vi "aim.vi"() -> (0 "rate":dbl)   [LabVIEW 2011]
doc: "Aims the turret at the selected target."
uses:
  vision data.ctl
  fg_typedef.ctl
  <vilib>/addons/control/pid/pid.llb/PID (DBL).vi
  <vilib>/addons/control/pid/NI_PID_pid.lvlib
  <vilib>/addons/control/pid/pid.llb/PID Control Input Filter (DBL).vi
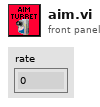
[diagram p1: front panel]
types:
  T1 = typedef "fg_typedef.ctl" = enum16{"Get", "Set"}
  T2 = typedef "vision data.ctl" = cluster{"x":dbl, "y":dbl, "area":dbl, "width":dbl, "height":dbl}
  T3 = cluster{"x":bool, "y":bool, "area":bool, "width":bool, "height":bool}
  T4 = typedef "WPI_EncoderDevRef.ctl" = cluster{"DevStatus":errorcluster, "EncoderIndex":T5, "CounterIndex":T6, "DistancePerCount":dbl, "Decoding Type":T7}
  T5 = typedef "FPGA_EncoderIdx.ctl" = enum8{"Enc 0", "Enc 1", "Enc 2", "Enc 3", "Invalid"}
  T6 = typedef "FPGA_CounterCtrSystemIndex.ctl" = enum8{"Ctr 0", "Ctr 1", "Ctr 2", "Ctr 3", "Ctr 4", "Ctr 5", "Ctr 6", "Ctr 7", "Invalid"}
  T7 = typedef "WPI_EncoderType.ctl" = enum16{"1x", "2x", "4x"}
  T8 = typedef "WPI_JoystickDevRef.ctl" = cluster{"Device":T9}
  T9 = typedef "WPI_JoystickDeviceEnum.ctl" = enum16{"USB 1", "USB 2", "USB 3", "USB 4", "Kinect 1", "Kinect 2"}
  T10 = cluster{"axis 1 (x)":dbl, "axis 2 (y)":dbl, "axis 3 (throttle)":dbl, "axis 4":dbl, "axis 5":dbl, "axis 6":dbl}
  T11 = cluster{"proportional gain (Kc)":dbl, "integral time (Ti, min)":dbl, "derivative time (Td, min)":dbl}
  T12 = cluster{dbl, "integral time (Ti, min)":dbl, "integral time (Ti, min)":dbl}
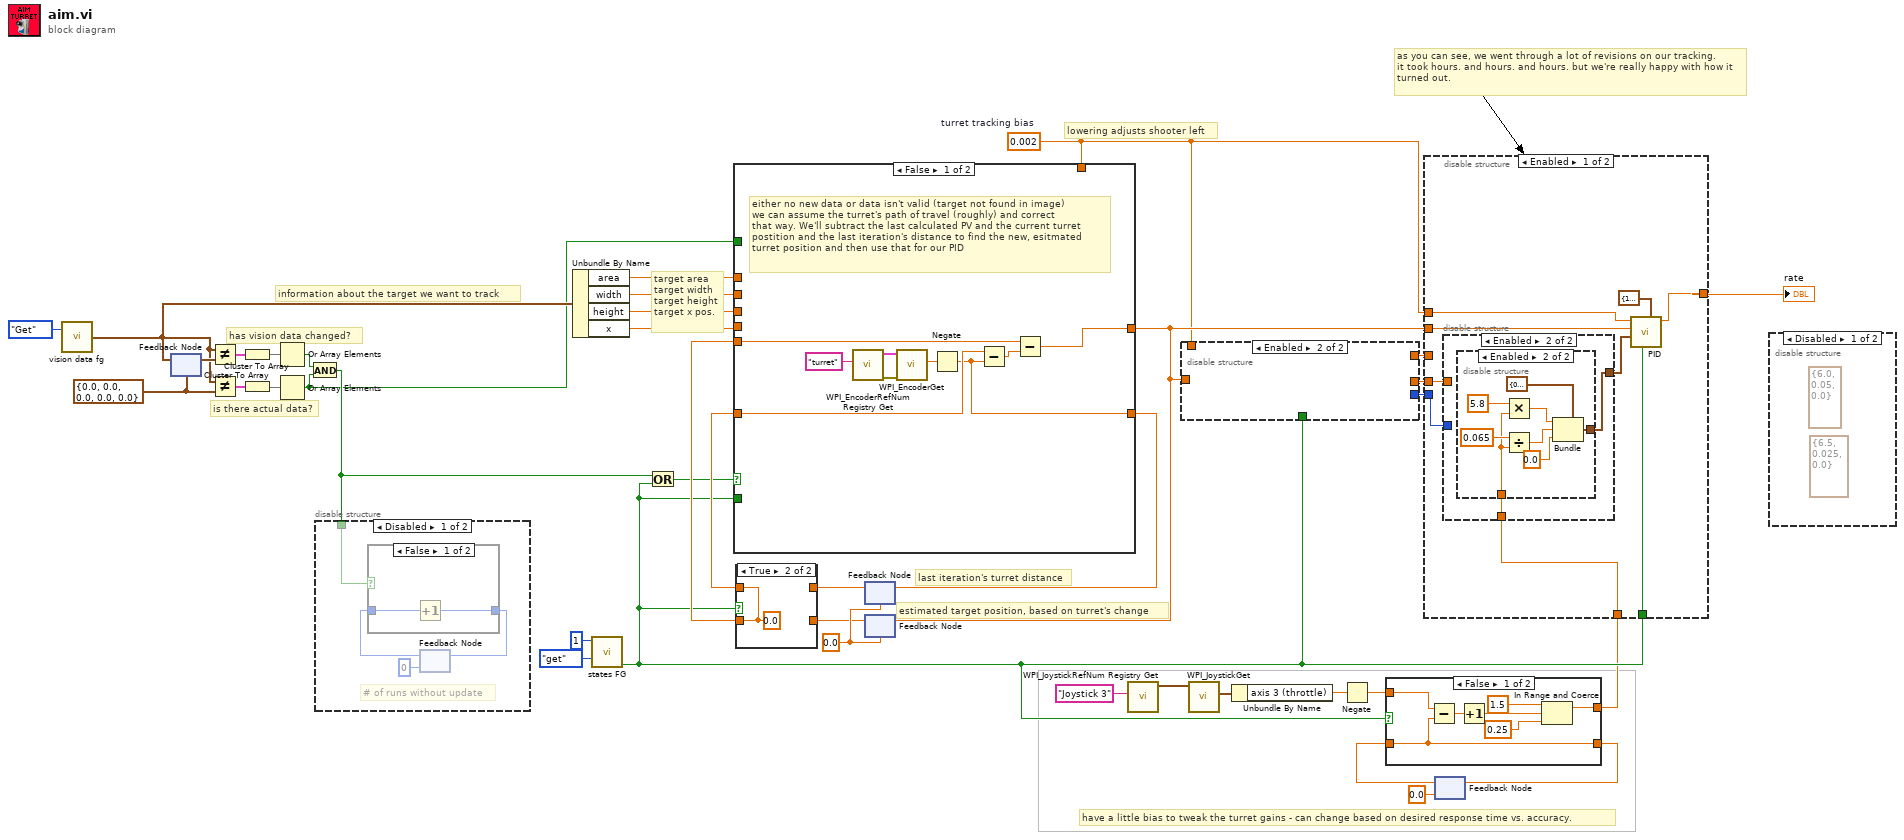
[diagram p0: block diagram]
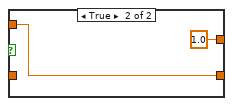
[diagram p2: hidden frame]
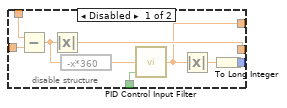
[diagram p3: hidden frame]
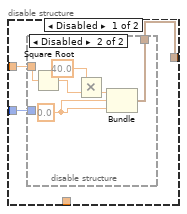
[diagram p4: hidden frame]
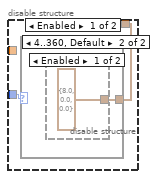
[diagram p5: hidden frame]
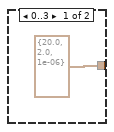
[diagram p6: hidden frame]
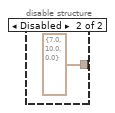
[diagram p7: hidden frame]
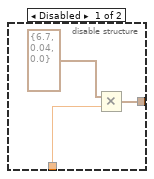
[diagram p8: hidden frame]
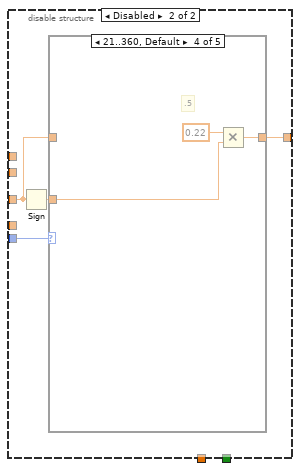
[diagram p9: hidden frame]
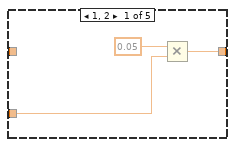
[diagram p10: hidden frame]
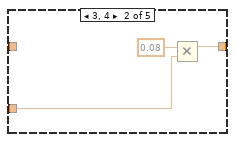
[diagram p11: hidden frame]
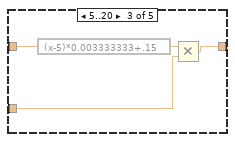
[diagram p12: hidden frame]
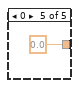
[diagram p13: hidden frame]
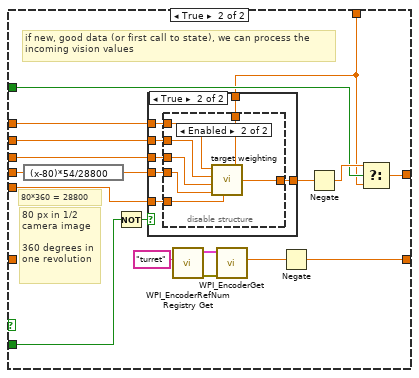
[diagram p15: hidden frame]
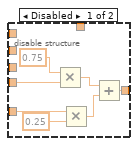
[diagram p17: hidden frame]
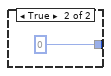
[diagram p19: hidden frame]
diagram:
  w19 = 0.002  # turret tracking bias
  w15 = T2 {"x"=0.0, "y"=0.0, "area"=0.0, "width"=0.0, "height"=0.0} ("Cluster")
  w30 = 0.0 ("x")
  # "information about the target we want to track"
  # "target area\ntarget width\ntarget height\ntarget x pos."
  # "as you can see, we went through a lot of revisions on our tracking.\nit took hours. and hours. and hours. but we're really happy with how it turned out."
  # "have a little bias to tweak the turret gains - can change based on desired response time vs. accuracy."
  # "estimated target position, based on turret's change"
  # "last iteration's turret distance"
  # "is there actual data?"
  # "has vision data changed?"
  # "lowering adjusts shooter left"
  n1 = call "vision data fg.vi"("Menu"=fg_typedef."Get") -> ("Data Output"=w34:T2)  [unwired: 1 in]
  n2 = feedback #1(w15) -> (w37:T2)
  n3 = feedback-in #1(w34) -> ()
  n4 = Not Equal?(x=w34, y=w37) -> (x != y?=w40:T3)
  n5 = Not Equal?(x=w34, y=w15) -> (x != y?=w38:T3)
  n6 = Cluster To Array(cluster=w40) -> (array=w39:bool[])
  n7 = Cluster To Array(cluster=w38) -> (array=w35:bool[])
  n8 = Or Array Elements(Boolean array=w39) -> (logical OR=w36:bool)
  n9 = Or Array Elements(Boolean array=w35) -> (logical OR=w16:bool)
  n10 = And(x=w36, y=w16) -> (x .and. y?=w33:bool)
  n11 = disable-structure shown="Disabled" {
    disable-tunnel: w33 -> [w41 _]
    frame Disabled {
      # "# of runs without update"
      n12 = feedback #2(0) -> (w43:i32)
      n13 = case shown="False" w41 {
        tunnel: [w45 0] -> w44
        tunnel: w43 -> [w46 _]
        frame False {
          n14 = Increment(x=w46) -> (x+1=w45:i32)
        }
        frame True {
        }
      }
      n15 = feedback-in #2(w44) -> ()
    }
    frame Enabled {
    }
  }
  n16 = Unbundle By Name(w34) -> ("area"=w13:dbl, "width"=w12:dbl, "height"=w11:dbl, "x"=w22:dbl)
  n17 = call "states FG.vi"("menu (get)"=enum16{"set", "get"}."get", "Loop ID"=1) -> ("first call?"=w7:bool)  [unwired: 6 in, 3 out]
  n18 = Or(x=w33, y=w7) -> (x .or. y?=w17:bool)
  n19 = feedback #3(w30) -> (w27:dbl)
  n20 = feedback #4(w30) -> (w26:dbl)
  n21 = case shown="True" w7 {
    tunnel: w27 -> [w48 _]
    tunnel: w26 -> [w49 _]
    tunnel: [w48 w50] -> w25
    tunnel: [w49 w50] -> w24
    frame False {
    }
    frame True {
      w50 = 0.0 ("x")
    }
  }
  n22 = case shown="False" w17 {
    tunnel: w22 -> [_ w77]
    tunnel: [w51 w68] -> w23
    tunnel: w24 -> [w52 w70]
    tunnel: [w53 w72] -> w31
    tunnel: w25 -> [w55 _]
    tunnel: w16 -> [_ w66]
    tunnel: w19 -> [_ w63]
    tunnel: w7 -> [_ w65]
    tunnel: w13 -> [_ w62]
    tunnel: w12 -> [_ w61]
    tunnel: w11 -> [_ w60]
    frame False {
      # "either no new data or data isn't valid (target not found in image)\nwe can assume the turret's path of travel (roughly) and correct\nthat way. We'll subtract the last calculated PV and the current turret \npostition and the last iteration's distance to find the new, esitmated\nturret position and then use that for our PID"
      n23 = call <vilib>:"WPI_EncoderRefNum Registry Get.vi"("refnum name"="turret") -> ("error out"=w58:errorcluster, "EncoderDevRef"=w57:T4)  [unwired: 9 in]
      n24 = call <vilib>:"WPI_EncoderGet.vi"("error in (no error)"=w58, "EncoderDevRef"=w57) -> ("Distance"=w56:dbl)  [unwired: 4 in, 5 out]
      n25 = Negate(x=w56) -> (-x=w53:dbl)
      n26 = Subtract(x=w55, y=w53) -> (x-y=w54:dbl)
      n27 = Subtract(x=w52, y=w54) -> (x-y=w51:dbl)
    }
    frame True {
      # "if new, good data (or first call to state), we can process the \nincoming vision values"
      # "80 px in 1/2 \ncamera image\n\n360 degrees in\none revolution"
      # "80*360 = 28800"
      n28 = expression code="(x-80)*54/28800"(w77) -> (w71:dbl)
      n29 = Not(x=w65) -> (.not. x?=w64:bool)
      n30 = case shown="True" w64 {
        tunnel: w71 -> [w78 w85]
        tunnel: w70 -> [_ w84]
        tunnel: [w78 w83] -> w69
        tunnel: w63 -> [_ w82]
        tunnel: w62 -> [_ w79]
        tunnel: w61 -> [_ w80]
        tunnel: w60 -> [_ w81]
        frame False {
        }
        frame True {
          n31 = disable-structure shown="Enabled" {
            disable-tunnel: w85 -> [w92 w96]
            disable-tunnel: w84 -> [w89 w97]
            disable-tunnel: [w86 w98] -> w83
            disable-tunnel: w82 -> [_ w99]
            disable-tunnel: w81 -> [_ w95]
            disable-tunnel: w80 -> [_ w94]
            disable-tunnel: w79 -> [_ w93]
            frame Disabled {
              n32 = Multiply(x=0.75 ("y"), y=w92) -> (x*y=w91:dbl)
              n33 = Multiply(x=w89, y=0.25) -> (x*y=w90:dbl)
              n34 = Add(x=w91, y=w90) -> (x+y=w86:dbl)
            }
            frame Enabled {
              n35 = call "target weighting.vi"("Area"=w93, "Width"=w94, "Height"=w95, "last offset"=w97, "offset"=w96, "bias"=w99) -> ("weighted offset"=w98:dbl)  [unwired: 2 in]
            }
          }
        }
      }
      n36 = call <vilib>:"WPI_EncoderRefNum Registry Get.vi"("refnum name"="turret") -> ("error out"=w75:errorcluster, "EncoderDevRef"=w74:T4)  [unwired: 9 in]
      n37 = call <vilib>:"WPI_EncoderGet.vi"("error in (no error)"=w75, "EncoderDevRef"=w74) -> ("Distance"=w73:dbl)  [unwired: 4 in, 5 out]
      n38 = Negate(x=w73) -> (-x=w72:dbl)
      n39 = Negate(x=w69) -> (-x=w67:dbl)
      n40 = Select(t=w67, s=w66, f=w63) -> (s? t:f=w68:dbl)
    }
  }
  n41 = feedback-in #3(w31) -> ()
  n42 = feedback-in #4(w23) -> ()
  n43 = call <vilib>:"WPI_JoystickRefNum Registry Get.vi"("refnum name"="Joystick 3") -> ("JoystickDevRef"=w9:T8)  [unwired: 9 in, 1 out]
  n44 = disable-structure shown="Enabled" {
    disable-tunnel: w23 -> [w108 _]
    disable-tunnel: [w107 _] -> w21
    disable-tunnel: [w105 _] -> w20
    disable-tunnel: w19 -> [w103 _]
    disable-tunnel: [w102 _] -> w18
    disable-tunnel: w7 -> [w100 _]
    frame Disabled {
      n45 = Subtract(x=w103, y=w108) -> (x-y=w106:dbl)
      n46 = Absolute Value(x=w106) -> (abs(x)=w105:dbl)
      n47 = expression code="-x*360"(w106) -> (w101:dbl)
      n48 = call-poly <vilib>:"PID Control Input Filter.vi"("reinitialize? (F)"=w100, "input"=w101) -> ("output"=w102:dbl)  [unwired: 3 in]
      n49 = Absolute Value(x=w102) -> (abs(x)=w104:dbl)
      n50 = To Long Integer(number=w104) -> (32bit integer=w107:i32)
    }
    frame Enabled {
    }
  }
  n51 = call <vilib>:"WPI_JoystickGet.vi"("JoystickDevRef"=w9) -> ("Axes"=w8:T10)  [unwired: 4 in, 2 out]
  n52 = Unbundle By Name(w8) -> ("axis 3 (throttle)"=w6:dbl)
  n53 = Negate(x=w6) -> (-x=w2:dbl)
  n54 = feedback #5(0.0 ("axis 3 (throttle)")) -> (w5:dbl)
  n55 = case shown="False" w7 {
    tunnel: w2 -> [w115 w117]
    tunnel: [w114 w117] -> w3
    tunnel: w5 -> [w114 _]
    tunnel: [w111 1.0 ("upper limit")] -> w1
    frame False {
      n56 = Subtract(x=w115, y=w114) -> (x-y=w110:dbl)
      n57 = Increment(x=w110) -> (x+1=w109:dbl)
      n58 = In Range and Coerce(upper limit=1.5, x=w109, lower limit=0.25) -> (coerced(x)=w111:dbl)  [unwired: 1 out]
    }
    frame True {
    }
  }
  n59 = disable-structure shown="Enabled" {
    disable-tunnel: [w124 w158] -> w32
    disable-tunnel: w23 -> [w123 _]
    disable-tunnel: w19 -> [w122 _]
    disable-tunnel: w7 -> [w121 _]
    disable-tunnel: w21 -> [w120 w156]
    disable-tunnel: w20 -> [w119 _]
    disable-tunnel: w18 -> [_ w155]
    disable-tunnel: w1 -> [w118 _]
    frame Enabled {
      n60 = disable-structure shown="Enabled" {
        disable-tunnel: [w129 w142] -> w125
        disable-tunnel: w120 -> [w128 _]
        disable-tunnel: w119 -> [w127 _]
        disable-tunnel: w118 -> [_ w143]
        frame Disabled {
          n61 = disable-structure shown="Disabled" {
            disable-tunnel: [w131 w138] -> w129
            disable-tunnel: w128 -> [w130 _]
            disable-tunnel: w127 -> [_ w139]
            frame Enabled {
              n62 = case shown="4..360, Default" w130 {
                tunnel: [T11 {"proportional gain (Kc)"=20.0, "integral time (Ti, min)"=2.0, "derivative time (Td, min)"=1e-06} ("PID gains") w133] -> w131
                frame 0..3 {
                }
                frame 4..360, Default {
                  n63 = disable-structure shown="Enabled" {
                    disable-tunnel: [T11 {"proportional gain (Kc)"=8.0, "integral time (Ti, min)"=0.0, "derivative time (Td, min)"=0.0} ("PID gains") T11 {"proportional gain (Kc)"=7.0, "integral time (Ti, min)"=10.0, "derivative time (Td, min)"=0.0} ("PID gains")] -> w133
                    frame Enabled {
                    }
                    frame Disabled {
                    }
                  }
                }
              }
            }
            frame Disabled {
              w141 = 0.0
              n64 = Square Root(x=w139) -> (sqrt(x)=w140:dbl)
              n65 = Multiply(x=40.0, y=w140) -> (x*y=w137:dbl)
              n66 = Bundle(w137, w141, w141) -> (w138:cluster{dbl, dbl, dbl})  [unwired: 1 in]
            }
          }
        }
        frame Enabled {
          n67 = disable-structure shown="Enabled" {
            disable-tunnel: w143 -> [w145 w147]
            disable-tunnel: [w144 w152] -> w142
            frame Disabled {
              n68 = Multiply(x=T11 {"proportional gain (Kc)"=6.7, "integral time (Ti, min)"=0.04, "derivative time (Td, min)"=0.0} ("PID gains"), y=w145) -> (x*y=w144:T11)
            }
            frame Enabled {
              n69 = Multiply(x=5.8 ("proportional gain (Kc)"), y=w147) -> (x*y=w153:dbl)
              n70 = Divide(x=0.065 ("integral time (Ti, min)"), y=w147) -> (x/y=w148:dbl)
              n71 = Bundle(cluster=T12 {0.0, "integral time (Ti, min)"=0.0, "integral time (Ti, min)"=0.0}, w153, "integral time (Ti, min)"=w148, "integral time (Ti, min)"=0.0) -> (w152:T12)
            }
          }
        }
      }
      n72 = call-poly <vilib>:"PID.vi"("reinitialize? (F)"=w121, "output range"=cluster{"output high":dbl, "output low":dbl} {"output high"=1.0, "output low"=-1.0}, "PID gains"=w125, "process variable"=w123, "setpoint"=w122) -> ("output"=w124:dbl)  [unwired: 5 in, 1 out]
    }
    frame Disabled {
      n73 = Sign(1:w155) -> (0:w157:dbl)
      n74 = case shown="21..360, Default" w156 {
        tunnel: [w161 w163 w165 w170 0.0] -> w158
        tunnel: w157 -> [w160 w162 w166 w169 _]
        tunnel: w155 -> [_ _ w168 _ _]
        frame 1, 2 {
          n75 = Multiply(x=0.05, y=w160) -> (x*y=w161:dbl)
        }
        frame 3, 4 {
          n76 = Multiply(x=0.08, y=w162) -> (x*y=w163:dbl)
        }
        frame 5..20 {
          n77 = expression code="(x-5)*0.003333333+.15"(w168) -> (w167:dbl)
          n78 = Multiply(x=w167, y=w166) -> (x*y=w165:dbl)
        }
        frame 21..360, Default {
          # ".5"
          n79 = Multiply(x=0.22, y=w169) -> (x*y=w170:dbl)
        }
        frame 0 {
        }
      }
    }
  }
  "rate" <- w32
  n80 = feedback-in #5(w3) -> ()
  n81 = disable-structure shown="Disabled" {
    frame Disabled {
      (unwired) T11 {"proportional gain (Kc)"=6.5, "integral time (Ti, min)"=0.025, "derivative time (Td, min)"=0.0} ("PID gains")
      (unwired) T11 {"proportional gain (Kc)"=6.0, "integral time (Ti, min)"=0.05, "derivative time (Td, min)"=0.0} ("PID gains")
    }
    frame Enabled {
    }
  }
